vi "Collision Detection global.vi"() -> ()   [LabVIEW 2016]
uses:
  <vilib>/Utility/miscctls.llb/LV3DPointTypeDef.ctl
  Traverse active parts.ctl
panel:
  in  "Fixed objects name":string="None"
  in  "Fixed objects octree resolution (model units)":sgl=100.0
  in  "Traverse active parts":T1=enum."XY and XYZ"
  in  "Auto-calc octree resolution":bool=TRUE
  in  "Traverse_XYZ look-out radius (model units)":sgl=100.0
  in  "Reset camera":bool=TRUE
  in  "Force reload geometry":bool
  in  "Draw octree leaf-node boxes":bool
  in  "Highlight tested triangles":bool=TRUE
  in  "Collision marker radius (mm)":sgl=25.0
  in  "Up Direction":T2={"X"=0.0, "Y"=0.0, "Z"=1.0}
  in  "Target":T2
  in  "Camera Position":T2={"X"=3500.0, "Y"=0.0, "Z"=1200.0}
  in  "Model name":string="MAGIC_London_Southbank_0_deg"
  in  "Model octree resolution (model units)":sgl=100.0
  in  "Tunnel octree resolution (model units)":sgl=100.0
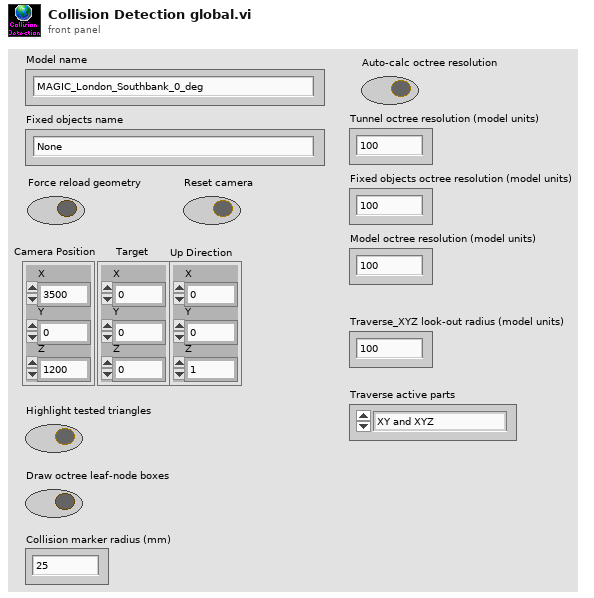
[diagram p1: front panel]
types:
  T1 = typedef "Traverse active parts.ctl" = enum16{"XYZ", "XY and XYZ", "X and XY and XYZ"}
  T2 = typedef "LV3DPointTypeDef.ctl" = cluster{"X":sgl, "Y":sgl, "Z":sgl}
diagram:
